vi "Data Loop.vi"(8 "Data":refnum<queue>, 10 "User Event in":refnum<user-event>, 11 "Data Loop Data":T1) -> (0 "error out":errorcluster)   [LabVIEW 2018]
uses:
  Type Defs/Data Loop Data.ctl
  Support/Message Queue/Message Cluster.ctl
  Support/Message Queue/Enqueue Message (Single).vi
  <vilib>/Utility/error.llb/Error Cluster From Error Code.vi
  <vilib>/ErrorRing/Error Ring.xnode
  Support/Message Queue/Message Queue.lvlib
  Support/User Event - Stop/User Event - Stop.lvlib
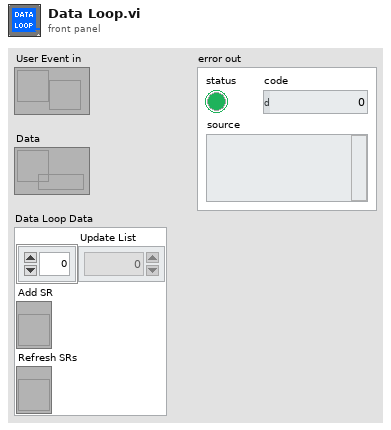
[diagram p1: front panel]
types:
  T1 = typedef "Data Loop Data.ctl" = cluster{"Update List":i32[], "Add SR":refnum<vi>, "Refresh SRs":refnum<vi>}
  T2 = typedef "SR Cluster.ctl" = cluster{"Color":u32, "SR Number":i32, "SR Status":T3, "SR Type":string, "Summary":string, "Last Updated":timestamp, "Service Level":string, "Days Open":dbl, "Creation Date":timestamp}
  T3 = typedef "SR Status.ctl" = enum16{"Caller Abandoned", "Created in Error", "Expired", "Forum Resolved AE", "Forum Resolved Customer", "IN WORK", "IN WORK Collab with AES", "IN WORK Collab with PSE", "IN WORK Collab with SE", "IN WORK Customer Added Note", "IN WORK Escalation", "IN WORK Wait on Customer", "Open", "Potentially Resolved", "Presumed Resolved", "RMA Approved for Return", "Resolved", "Passed Off"}
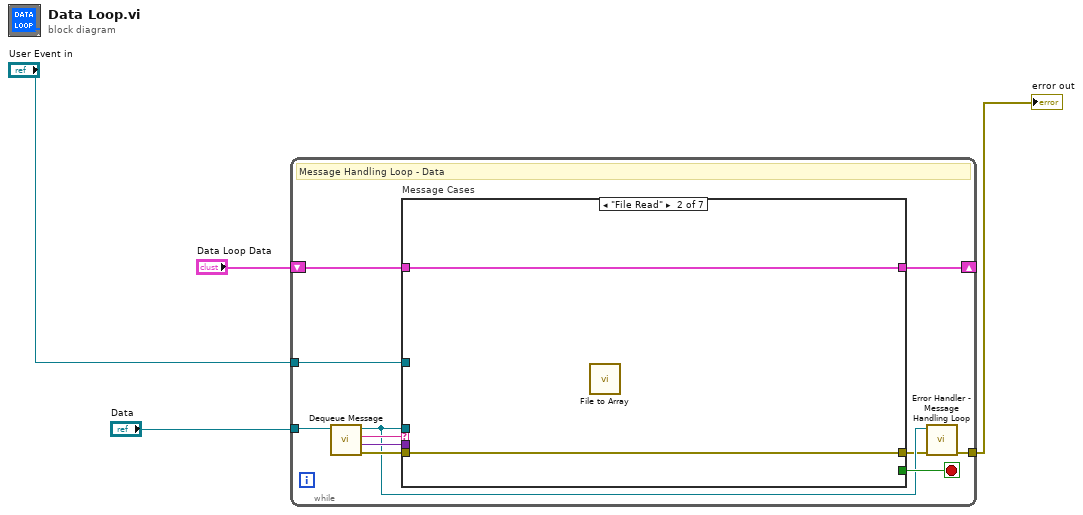
[diagram p0: block diagram]
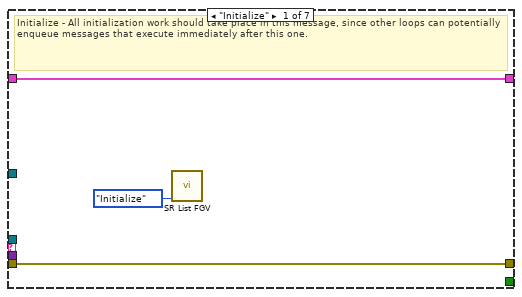
[diagram p2: hidden frame]
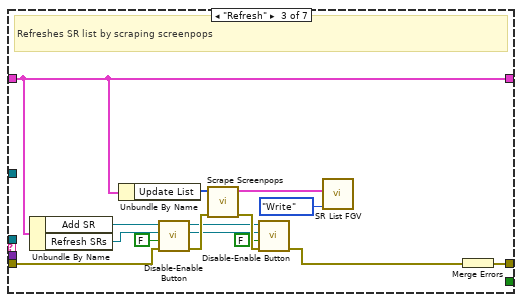
[diagram p3: hidden frame]
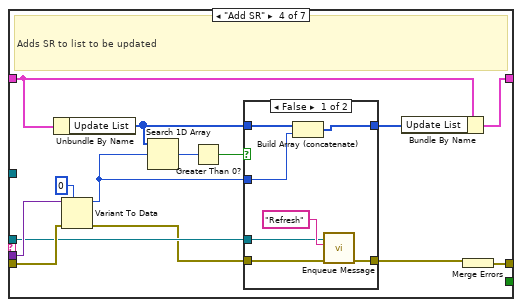
[diagram p4: hidden frame]
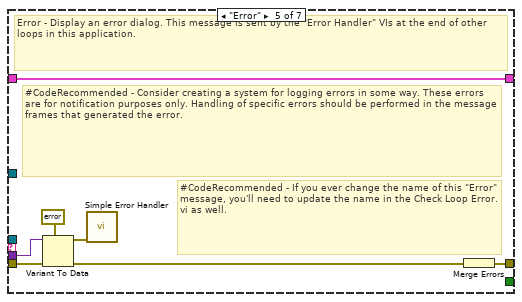
[diagram p6: hidden frame]
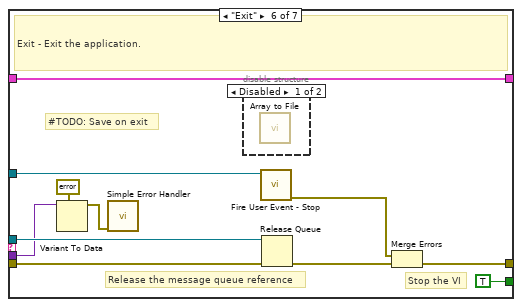
[diagram p7: hidden frame]
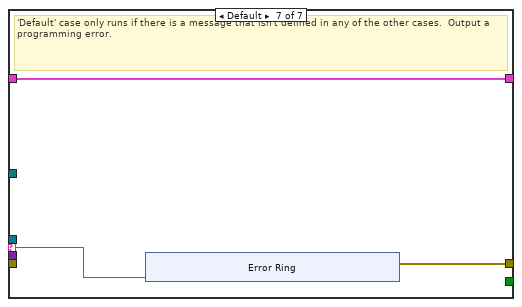
[diagram p9: hidden frame]
diagram:
  n1 = while {
    tunnel: "Data" -> [w11]
    tunnel: [w9] -> w3
    tunnel: "User Event in" -> [w7]
    shift-right: [w5] -> _
    shift-left: "Data Loop Data" -> [w6]
    stop <- w15 stop-if-true
    # "Message Handling Loop - Data"
    n2 = call "Dequeue Message.vi"("Message Queue"=w11) -> ("error out"=w14:errorcluster, "Message Data"=w12:variant, "Message"=w13:string, "dup Message Queue"=w10:refnum<queue>)  [unwired: 7 in]
    n3 = case "Message Cases" shown="\"File Read\"" w13 {
      selector: w13 -> [_ _ _ _ _ _ w78]
      tunnel: w10 -> [_ _ _ w38 _ w76 _]
      tunnel: w14 -> [w17 w20 w31 w45 w65 w71 _]
      tunnel: [w17 w20 w35 w49 w60 w73 w79] -> w8
      tunnel: [_ _ _ _ _ TRUE _] -> w15
      tunnel: w12 -> [_ _ _ w46 w64 w68 _]
      tunnel: w7 -> [_ _ _ _ _ w67 _]
      tunnel: w6 -> [w18 w19 w29 w48 w59 w66 w77]
      tunnel: [w18 w19 w29 w47 w59 w66 w77] -> w5
      frame "Initialize" {
        # "Initialize - All initialization work should take place in this message, since other loops can potentially enqueue messages that execute immediately after this one."
        n4 = call "SR List FGV.vi"("Operation"=enum16{"Initialize", "Write", "Read", "Clear"}."Initialize") -> ()  [unwired: 9 in, 2 out]
      }
      frame "File Read" {
        n5 = call "File to Array.vi"() -> ()  [unwired: 9 in, 3 out]
      }
      frame "Refresh" {
        # "Refreshes SR list by scraping screenpops"
        n6 = Unbundle By Name(w29) -> ("Add SR"=w33:refnum<vi>, "Refresh SRs"=w32:refnum<vi>)
        n7 = Unbundle By Name(w29) -> ("Update List"=w34:i32[])
        n8 = call "Disable-Enable Button.vi"("error in"=w31, "Enabled?"=FALSE, "Refresh SRs in"=w32, "Add SR in"=w33) -> ("error out"=w30:errorcluster, "Refresh SRs out"=w25:refnum<vi>, "Add SR out"=w26:refnum<vi>)  [unwired: 5 in]
        n9 = call "Scrape Screenpops.vi"("error in"=w30, "SR number list in"=w34) -> ("error out"=w27:errorcluster, "sr clusters out"=w21:T2[])  [unwired: 8 in]
        n10 = call "Disable-Enable Button.vi"("error in"=w27, "Enabled?"=FALSE, "Refresh SRs in"=w25, "Add SR in"=w26) -> ("error out"=w24:errorcluster)  [unwired: 5 in, 2 out]
        n11 = call "SR List FGV.vi"("Operation"=enum16{"Initialize", "Write", "Read", "Clear"}."Write", "list in"=w21) -> ()  [unwired: 8 in, 2 out]
        n12 = Merge Errors(w24) -> (w35:errorcluster)
      }
      frame "Add SR" {
        # "Adds SR to list to be updated"
        n13 = Unbundle By Name(w48) -> ("Update List"=w40:i32[])
        n14 = Variant To Data(error in=w45, type=0, Variant=w46) -> (data=w39:i32, error out=w36:errorcluster)
        n15 = Search 1D Array(1D array=w40, element=w39) -> (index of element=w43:i32)  [unwired: 1 in]
        n16 = Greater Than 0?(x=w43) -> (x > 0?=w42:bool)
        n17 = case shown="False" w42 {
          tunnel: [w55 w58] -> w41
          tunnel: w40 -> [w56 w58]
          tunnel: w39 -> [w54 _]
          tunnel: w38 -> [w52 _]
          tunnel: [w51 w57] -> w37
          tunnel: w36 -> [w50 w57]
          frame False {
            n18 = Build Array (concatenate)(w56, w54) -> (w55:i32[])
            n19 = call-poly "Enqueue Message.vi"("error in (no error)"=w50, "Message"="Refresh", "Message Queue"=w52) -> ("error out"=w51:errorcluster)  [unwired: 7 in, 1 out]
          }
          frame True {
          }
        }
        n20 = Bundle By Name(cluster=w48, "Update List"=w41) -> (w47:T1)
        n21 = Merge Errors(w37) -> (w49:errorcluster)
      }
      frame "Error" {
        # "#CodeRecommended - If you ever change the name of this \"Error\" message, you'll need to update the name in the Check Loop Error.vi as well."
        # "#CodeRecommended - Consider creating a system for logging errors in some way. These errors are for notification purposes only. Handling of specific errors should be performed in the message frames that generated the error."
        # "Error - Display an error dialog. This message is sent by the \"Error Handler\" VIs at the end of other loops in this application."
        n22 = Variant To Data(error in=w65, type=errorcluster {"status"=FALSE, "code"=0, "source"=""} ("error constant"), Variant=w64) -> (data=w62:errorcluster, error out=w61:errorcluster)
        n23 = call <vilib>:"Simple Error Handler.vi"("error in (no error)"=w62) -> ()  [unwired: 4 in, 5 out]
        n24 = Merge Errors(w61) -> (w60:errorcluster)
      }
      frame "Exit" {
        # "#TODO: Save on exit"
        # "Stop the VI"
        # "Release the message queue reference"
        # "Exit - Exit the application."
        n25 = Variant To Data(type=errorcluster {"status"=FALSE, "code"=0, "source"=""} ("error constant"), Variant=w68) -> (data=w69:errorcluster)  [unwired: 1 in, 1 out]
        n26 = call <vilib>:"Simple Error Handler.vi"("error in (no error)"=w69) -> ()  [unwired: 4 in, 5 out]
        n27 = disable-structure shown="Disabled" {
          frame Disabled {
            n28 = call "Array to File.vi"() -> ()  [unwired: 10 in, 2 out]
          }
          frame Enabled {
          }
        }
        n29 = call "Fire User Event - Stop.vi"("User Event - Stop"=w67) -> ("error out"=w72:errorcluster)  [unwired: 10 in]
        n30 = Release Queue(queue=w76, error in (no error)=w71) -> (error out=w74:errorcluster)  [unwired: 1 in, 2 out]
        n31 = Merge Errors(w72, w74) -> (w73:errorcluster)
      }
      frame Default {
        # "'Default' case only runs if there is a message that isn't defined in any of the other cases.  Output a programming error."
        n32 = xnode "Error Ring"("parameter 0"=w78) -> ("error out"=w79:errorcluster)
      }
    }
    n33 = call "Error Handler - Message Handling Loop.vi"("error in (no error)"=w8, "Message Queue"=w10) -> ("dup error in"=w9:errorcluster)  [unwired: 8 in, 1 out]
  }
  "error out" <- w3
